vi "Benchmarking Time Delay.vi"() -> ()   [LabVIEW 2014]
panel:
  in  "stop":bool
  out "Actual Delay (ms)":dbl
  out "Count":i32
  in  "N":i32
  # "Benchmarking Time Delay"
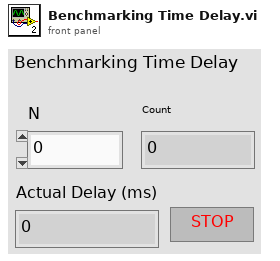
[diagram p1: front panel]
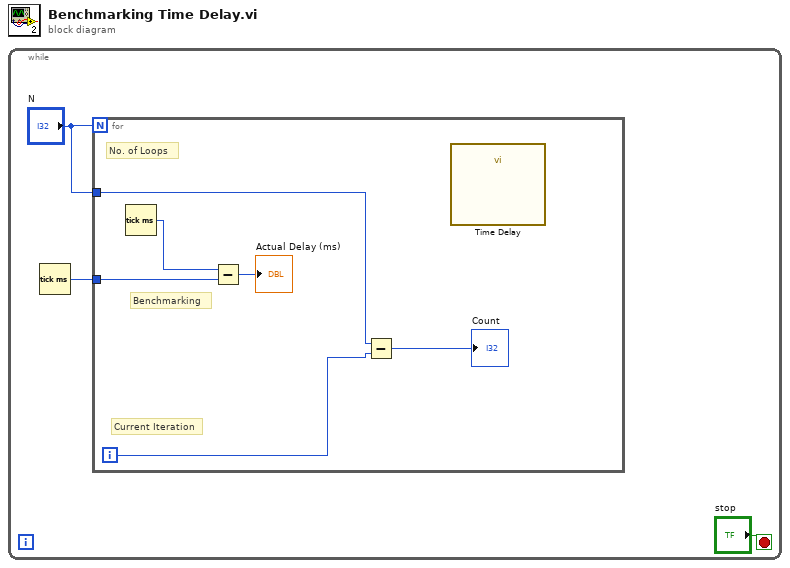
[diagram p0: block diagram]
diagram:
  n1 = while {
    stop <- "stop" stop-if-true
    n2 = Tick Count (ms)() -> (millisecond timer value=w3:u32)
    n3 = for {
      N: "N" -> [_]
      tunnel: w3 -> [w8]
      tunnel: "N" -> [w6]
      i -> [w4]
      # "Benchmarking"
      # "Current Iteration"
      # "No. of Loops"
      n4 = Tick Count (ms)() -> (millisecond timer value=w7:u32)
      n5 = Subtract(x=w7, y=w8) -> (x-y=→"Actual Delay (ms)":u32)
      n6 = Subtract(x=w6, y=w4) -> (x-y=→"Count":i32)
      n7 = call "Time Delay"() -> ()  [unwired: 11 in, 1 out]
    }
  }
